vi "蓄电池配置同步 (子VI).vi"   [LabVIEW 2016, in "环境动力监测库.lvlib"]
uses:
  <vilib>/Utility/config.llb/NI_LVConfig.lvlib
types:
  T1 = cluster{"baud rate (bps)":u32, "stop bits":u16, "parity":u16, "flow control":u16, "timeout":u32, "retries":i32}
  T2 = cluster{"监测项描述:输出":string, "连接方式":enum16{"串口", "TCP"}, "端口":string, "IP address:":string, "Port:":string, "站号":u64, "传感器型号":string, "波特率":u64, "data bits":u64, "停止位":u16, "奇偶校验":u16}
  T3 = typedef "NI_LVConfig.lvlib/Config Data RefNum.ctl" = refnum<k1>
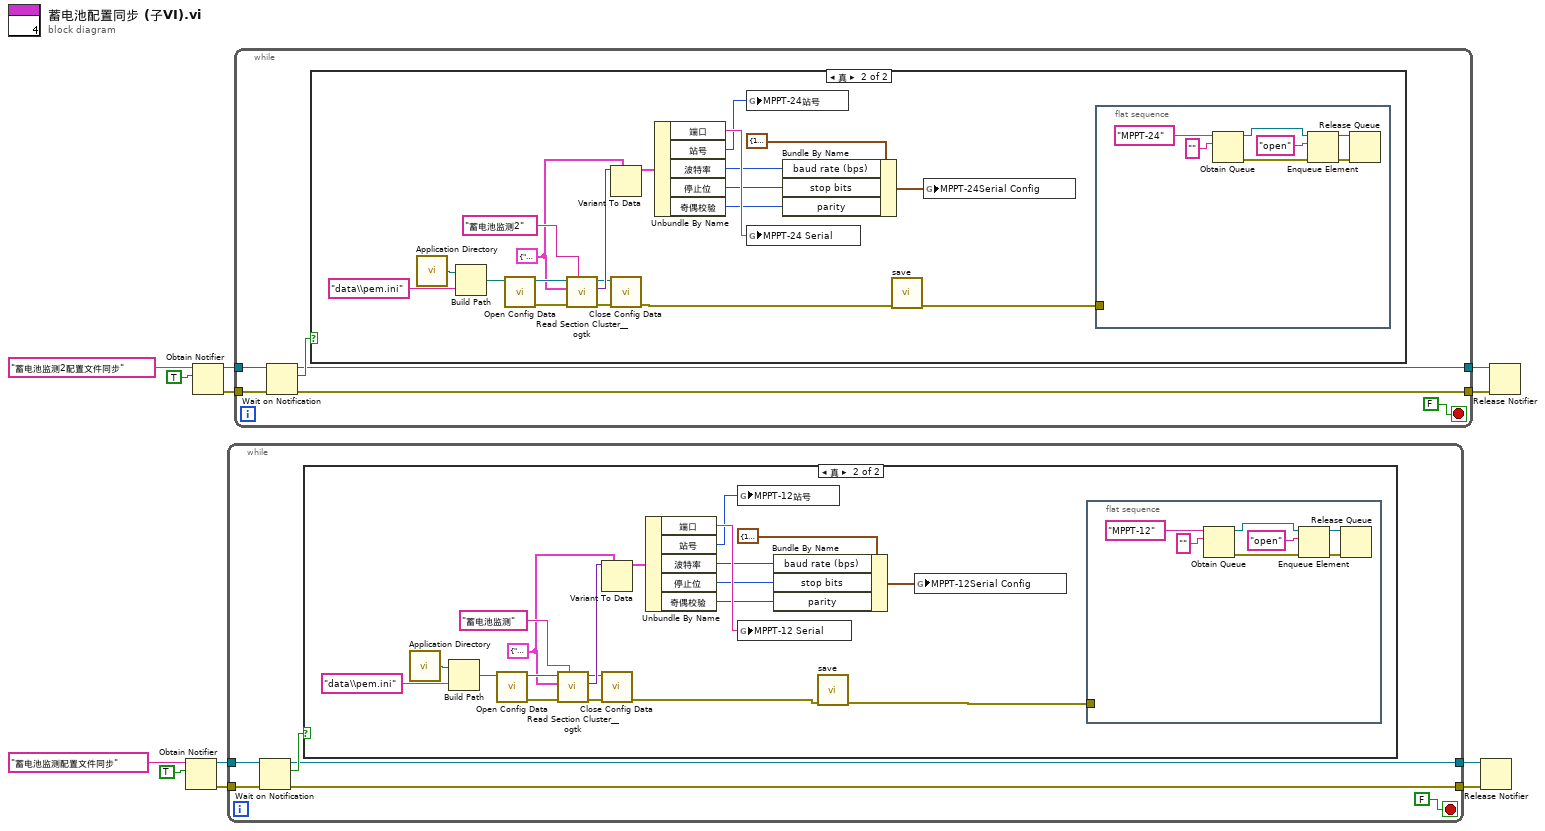
[diagram p0: block diagram]
diagram:
  n1 = Obtain Notifier(name (unnamed)="蓄电池监测配置文件同步" ("名称（未命名）"), notification data type=TRUE) -> (notifier out=w4:refnum<notifier>, error out=w3:errorcluster)  [unwired: 2 in, 1 out]
  n2 = Obtain Notifier(name (unnamed)="蓄电池监测2配置文件同步" ("名称（未命名）"), notification data type=TRUE) -> (notifier out=w9:refnum<notifier>, error out=w10:errorcluster)  [unwired: 2 in, 1 out]
  n3 = while {
    tunnel: w4 -> [w18]
    tunnel: w3 -> [w17]
    tunnel: [w14] -> w2
    tunnel: [w13] -> w1
    stop <- FALSE stop-if-true
    n4 = Wait on Notification(notifier=w18, error in (no error)=w17) -> (notifier out=w14:refnum<notifier>, notification=w16:bool, error out=w13:errorcluster)  [unwired: 2 in, 1 out]
    n5 = case shown="真" w16 {
      frame False {
      }
      frame True {
        w28 = T2 {"监测项描述:输出"="", "连接方式"=enum."串口", "端口"="", "IP address:"="", "Port:"="", "站号"=19200, "传感器型号"="", "波特率"=19200, "data bits"=8, "停止位"=10, "奇偶校验"=0} ("输入簇")
        n6 = call <vilib>:"Application Directory.vi"() -> ("Application Directory"=w32:path)
        n7 = Build Path(base path=w32, name or relative path="data\\pem.ini" ("名称或相对路径")) -> (appended path=w31:path)
        n8 = call <vilib>:"Open Config Data.vi"("configuration file path"=w31) -> ("error out"=w30:errorcluster, "refnum"=w29:T3)  [unwired: 8 in, 1 out]
        n9 = call <userlib>:"Read Section Cluster__ogtk.vi"("section (optional)"="蓄电池监测", "error in (no error)"=w30, "Section Formatted Cluster Type"=w28, "refnum"=w29) -> ("error out"=w36:errorcluster, "Section Formatted Cluster"=w37:variant, "dup refnum"=w35:T3)  [unwired: 3 in, 2 out]
        n10 = Variant To Data(type=w28, Variant=w37) -> (data=w38:T2)  [unwired: 1 in, 1 out]
        n11 = call <vilib>:"Close Config Data.vi"("error in (no error)"=w36, "refnum"=w35) -> ("error out"=w20:errorcluster)  [unwired: 8 in, 1 out]
        n12 = Unbundle By Name(w38) -> ("端口"=w27:string, "站号"=w24:u64, "波特率"=w23:u64, "停止位"=w22:u16, "奇偶校验"=w21:u16)
        n13 = global write "断电保存全局变量.vi" "MPPT-12站号"(w24) -> ()
        n14 = global write "断电保存全局变量.vi" "MPPT-12 Serial"(w27) -> ()
        n15 = Bundle By Name(cluster=T1 {"baud rate (bps)"=115200, "stop bits"=10, "parity"=0, "flow control"=0, "timeout"=1000, "retries"=1} ("MPPT-24Serial Config"), "baud rate (bps)"=w23, "stop bits"=w22, "parity"=w21) -> (w25:T1)
        n16 = call "save.vi"("error in (no error)"=w20) -> ("error out"=w19:errorcluster)  [unwired: 10 in]
        n17 = global write "断电保存全局变量.vi" "MPPT-12Serial Config"(w25) -> ()
        n18 = flat-sequence {
          tunnel: w19 -> [_]
          frame #0 {
            n19 = Obtain Queue(name (unnamed)="MPPT-12" ("名称（未命名）"), element data type="") -> (queue out=w41:refnum<queue>, error out=w42:errorcluster)  [unwired: 3 in, 1 out]
            n20 = Enqueue Element(queue=w41, element="open", error in (no error)=w42) -> (queue out=w44:refnum<queue>, error out=w45:errorcluster)  [unwired: 1 in, 1 out]
            n21 = Release Queue(queue=w44, error in (no error)=w45) -> ()  [unwired: 1 in, 3 out]
          }
        }
      }
    }
  }
  n22 = while {
    tunnel: w9 -> [w51]
    tunnel: w10 -> [w50]
    tunnel: [w47] -> w11
    tunnel: [w46] -> w12
    stop <- FALSE stop-if-true
    n23 = Wait on Notification(notifier=w51, error in (no error)=w50) -> (notifier out=w47:refnum<notifier>, notification=w49:bool, error out=w46:errorcluster)  [unwired: 2 in, 1 out]
    n24 = case shown="真" w49 {
      frame False {
      }
      frame True {
        w61 = T2 {"监测项描述:输出"="", "连接方式"=enum."串口", "端口"="", "IP address:"="", "Port:"="", "站号"=19200, "传感器型号"="", "波特率"=19200, "data bits"=8, "停止位"=10, "奇偶校验"=0} ("输入簇")
        n25 = call <vilib>:"Application Directory.vi"() -> ("Application Directory"=w65:path)
        n26 = Build Path(base path=w65, name or relative path="data\\pem.ini" ("名称或相对路径")) -> (appended path=w64:path)
        n27 = call <vilib>:"Open Config Data.vi"("configuration file path"=w64) -> ("error out"=w63:errorcluster, "refnum"=w62:T3)  [unwired: 8 in, 1 out]
        n28 = call <userlib>:"Read Section Cluster__ogtk.vi"("section (optional)"="蓄电池监测2", "error in (no error)"=w63, "Section Formatted Cluster Type"=w61, "refnum"=w62) -> ("error out"=w69:errorcluster, "Section Formatted Cluster"=w70:variant, "dup refnum"=w68:T3)  [unwired: 3 in, 2 out]
        n29 = Variant To Data(type=w61, Variant=w70) -> (data=w71:T2)  [unwired: 1 in, 1 out]
        n30 = call <vilib>:"Close Config Data.vi"("error in (no error)"=w69, "refnum"=w68) -> ("error out"=w53:errorcluster)  [unwired: 8 in, 1 out]
        n31 = Unbundle By Name(w71) -> ("端口"=w60:string, "站号"=w57:u64, "波特率"=w56:u64, "停止位"=w55:u16, "奇偶校验"=w54:u16)
        n32 = global write "断电保存全局变量.vi" "MPPT-24站号"(w57) -> ()
        n33 = global write "断电保存全局变量.vi" "MPPT-24 Serial"(w60) -> ()
        n34 = Bundle By Name(cluster=T1 {"baud rate (bps)"=115200, "stop bits"=10, "parity"=0, "flow control"=0, "timeout"=1000, "retries"=1} ("MPPT-24Serial Config"), "baud rate (bps)"=w56, "stop bits"=w55, "parity"=w54) -> (w58:T1)
        n35 = call "save.vi"("error in (no error)"=w53) -> ("error out"=w52:errorcluster)  [unwired: 10 in]
        n36 = global write "断电保存全局变量.vi" "MPPT-24Serial Config"(w58) -> ()
        n37 = flat-sequence {
          tunnel: w52 -> [_]
          frame #0 {
            n38 = Obtain Queue(name (unnamed)="MPPT-24" ("名称（未命名）"), element data type="") -> (queue out=w74:refnum<queue>, error out=w75:errorcluster)  [unwired: 3 in, 1 out]
            n39 = Enqueue Element(queue=w74, element="open", error in (no error)=w75) -> (queue out=w77:refnum<queue>, error out=w78:errorcluster)  [unwired: 1 in, 1 out]
            n40 = Release Queue(queue=w77, error in (no error)=w78) -> ()  [unwired: 1 in, 3 out]
          }
        }
      }
    }
  }
  n41 = Release Notifier(notifier=w2, error in (no error)=w1) -> ()  [unwired: 1 in, 3 out]
  n42 = Release Notifier(notifier=w11, error in (no error)=w12) -> ()  [unwired: 1 in, 3 out]
